vi "Load Components.vi"(8 "error in (no error)":errorcluster) -> (0 "error out":errorcluster, 3 "Components":refnum<class "Component.lvclass">[](array[class]))   [LabVIEW 2019, in "DSF System Explorer.lvlib"]
uses:
  DSF System Explorer.lvlib
  DSF Core.lvlibp/Classes/Component/Component.lvclass
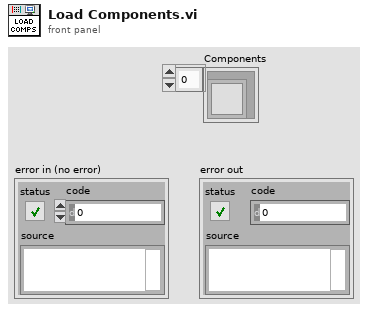
[diagram p1: front panel]
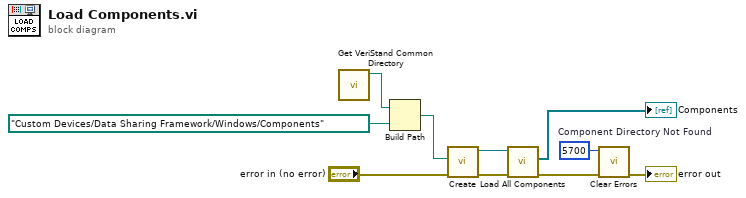
[diagram p0: block diagram]
diagram:
  w1 = 5700  # Component Directory Not Found
  n1 = call "Get VeriStand Common Directory.vi"() -> ("common directory"=w9:path)  [unwired: 11 in]
  n2 = Build Path(base path=w9, name or relative path=path "Custom Devices/Data Sharing Framework/Windows/Components") -> (appended path=w7:path)
  n3 = call "Create.vi"("error in (no error)"="error in (no error)", "components directory"=w7) -> ("error out"=w5:errorcluster, "Component Loader out"=w6:refnum<class "Component Loader.lvclass">)  [unwired: 8 in]
  n4 = call "Load All Components.vi"("error in (no error)"=w5, "Component Loader in"=w6) -> ("error out"=w3:errorcluster, "Components"=→"Components":refnum<class "Component.lvclass">[])  [unwired: 7 in, 1 out]
  n5 = call <vilib>:"Clear Errors.vi"("error in (no error)"=w3, "specific error code to clear (0: all)"=w1) -> ("error out"=→"error out":errorcluster)  [unwired: 4 in, 1 out]
